vi "Calcu_Surface Plate.vi"(7 "Condition":string[][](array[string]), 8 "Data in":string[][](array[string])) -> (0 "행크기":u32, 2 "배열":string[][](array[string]), 3 "Data out":string[][](array[string]))   [LabVIEW 2020]
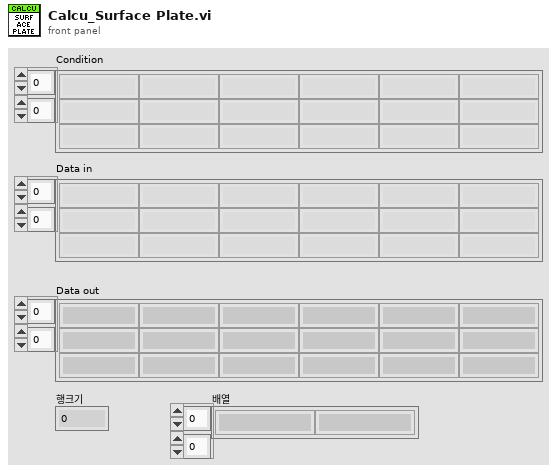
[diagram p1: front panel]
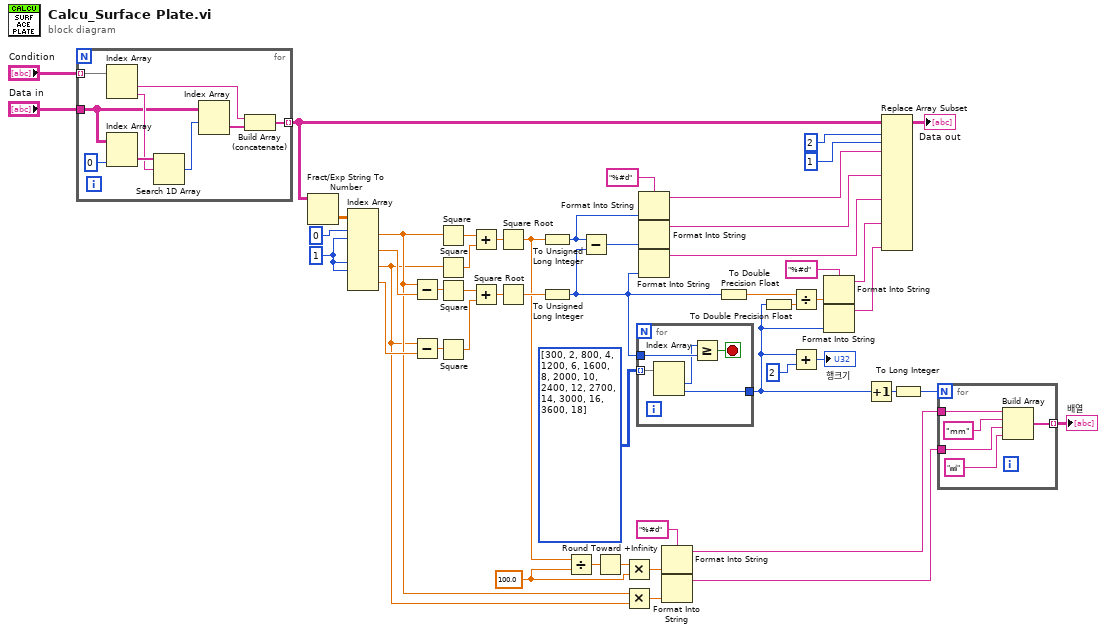
[diagram p0: block diagram]
diagram:
  w11 = 100.0 ("y")
  w7 = "%#d" ("포맷 문자열")
  w18 = "%#d" ("포맷 문자열")
  w23 = "%#d" ("포맷 문자열")
  w29 = 1 ("인덱스 (행)")
  n1 = for {
    tunnel: "Data in" -> [w56]
    tunnel: "Condition" -> [w58] mode=indexing
    tunnel: [w53] -> w49 mode=indexing
    n2 = Index Array(array=w58) -> (element #1=w52:string, element #2=w57:string)  [unwired: 2 in]
    n3 = Index Array(array=w56, index (col)=0 ("비활성화된 인덱스 (열)")) -> (element=w59:string[])  [unwired: 1 in]
    n4 = Search 1D Array(1D array=w59, element=w57) -> (index of element=w55:i32)  [unwired: 1 in]
    n5 = Index Array(array=w56, index (row)=w55) -> (element=w54:string[])  [unwired: 1 in]
    n6 = Build Array (concatenate)(w52, w54) -> (w53:string[])
  }
  n7 = Fract/Exp String To Number(string=w49) -> (number=w32:dbl[][])  [unwired: 3 in, 1 out]
  n8 = Index Array(array=w32, index (row) #1=0 ("인덱스 (행)"), index (col) #1=w29, index (row) #3=w29, index (col) #3=w29) -> (element #1=w10:dbl, element #2=w30:dbl, element #3=w9:dbl, element #4=w28:dbl)  [unwired: 4 in]
  n9 = Subtract(x=w10, y=w30) -> (x-y=w34:dbl)
  n10 = Subtract(x=w9, y=w28) -> (x-y=w33:dbl)
  n11 = Square(x=w10) -> (x^2=w40:dbl)
  n12 = Square(x=w9) -> (x^2=w39:dbl)
  n13 = Square(x=w34) -> (x^2=w35:dbl)
  n14 = Square(x=w33) -> (x^2=w36:dbl)
  n15 = Add(x=w40, y=w39) -> (x+y=w38:dbl)
  n16 = Add(x=w35, y=w36) -> (x+y=w37:dbl)
  n17 = Square Root(x=w38) -> (sqrt(x)=w15:dbl)
  n18 = Square Root(x=w37) -> (sqrt(x)=w19:dbl)
  n19 = To Unsigned Long Integer(number=w15) -> (unsigned 32bit integer=w27:u32)
  n20 = To Unsigned Long Integer(number=w19) -> (unsigned 32bit integer=w5:u32)
  n21 = Divide(x=w15, y=w11) -> (x/y=w14:dbl)
  n22 = Subtract(x=w27, y=w5) -> (x-y=w25:u32)
  n23 = Round Toward +Infinity(x=w14) -> (ceil(x): smallest int >= x=w13:dbl)
  n24 = Multiply(x=w13, y=w11) -> (x*y=w12:dbl)
  n25 = Multiply(x=w10, y=w9) -> (x*y=w8:dbl)
  n26 = for {
    tunnel: u32[][] [[300, 2], [800, 4], [1200, 6], [1600, 8], [2000, 10], [2400, 12], [2700, 14], [3000, 16], [3600, 18]] -> [w65] mode=indexing
    tunnel: w5 -> [w64]
    tunnel: [w61] -> w3
    stop <- w62 stop-if-true
    n27 = Index Array(array=w65) -> (element #1=w63:u32, element #2=w61:u32)  [unwired: 2 in]
    n28 = Greater Or Equal?(x=w63, y=w64) -> (x >= y?=w62:bool)
  }
  n29 = Format Into String(format string=w23, w27) -> (resulting string=w16:string)  [unwired: 2 in, 1 out]
  n30 = Format Into String(format string=w23, w25) -> (resulting string=w24:string)  [unwired: 2 in, 1 out]
  n31 = Format Into String(format string=w23, w5) -> (resulting string=w22:string)  [unwired: 2 in, 1 out]
  n32 = Format Into String(format string=w7, w12) -> (resulting string=w47:string)  [unwired: 2 in, 1 out]
  n33 = Format Into String(format string=w7, w8) -> (resulting string=w46:string)  [unwired: 2 in, 1 out]
  n34 = To Double Precision Float(number=w5) -> (double precision float=w4:dbl)
  n35 = To Double Precision Float(number=w3) -> (double precision float=w2:dbl)
  n36 = Divide(x=w4, y=w2) -> (x/y=w1:dbl)
  n37 = Add(x=w3, y=u32 2) -> (x+y=→"행크기":u32)
  n38 = Format Into String(format string=w18, w1) -> (resulting string=w21:string)  [unwired: 2 in, 1 out]
  n39 = Format Into String(format string=w18, w3) -> (resulting string=w17:string)  [unwired: 2 in, 1 out]
  n40 = Increment(x=w3) -> (x+1=w45:u32)
  n41 = Replace Array Subset(array=w49, new element #1=w16, index (row) #1=2 ("인덱스 (행)"), index (col) #1=1 ("비활성화된 인덱스 (열)"), new element #2=w24, new element #3=w22, new element #4=w21, new element #5=w17) -> (→"Data out":string[][])  [unwired: 8 in]
  n42 = To Long Integer(number=w45) -> (32bit integer=w44:i32)
  n43 = for {
    N: w44 -> [_]
    tunnel: [w70] -> w48 mode=indexing
    tunnel: w47 -> [w68]
    tunnel: w46 -> [w67]
    n44 = Build Array(w68, "mm", w67, "㎟") -> (w70:string[])
  }
  "배열" <- w48
